vi "Histogram Matching.vi"() -> ()   [LabVIEW 2014]
doc: "Use this template to build a VI to use as a subVI."
uses:
  <vilib>/vision/NI_Vision_Development_Module.lvlib
panel:
  out "H-Target":T1(graph)
  out "Target":T2(plugin-control)
  out "H-Dst":T1(graph)
  out "Dst":T2(plugin-control)
  out "H-Src":T1(graph)
  out "Src":T2(plugin-control)
  # ":: MVi Framework V1.0 ::\nAuthor:Gaoke Yang\nEmail: gaoke.yang@yahoo.com\nWeb: www.mvicontrol.com\nCopyright (C) 2015, MVI Technologies All Rights Reserved"
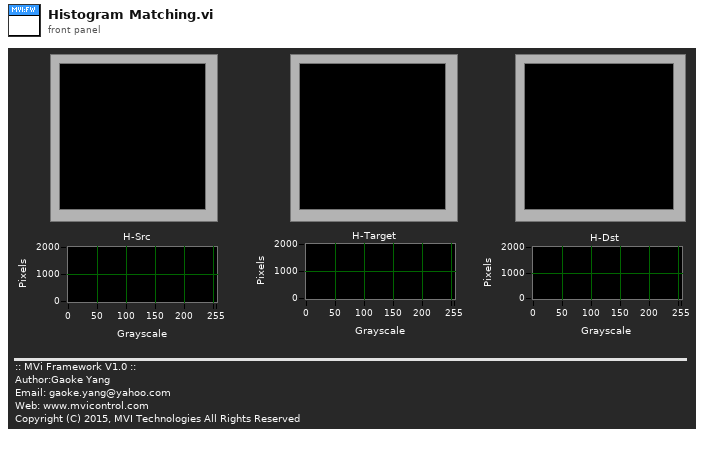
[diagram p1: front panel]
types:
  T1 = cluster{"Starting Value":sgl, "Incremental Value":sgl, "Histogram":u32[]}
  T2 = typedef "IMAQ Image.ctl" = refnum<image>
  T3 = typedef "Image Type" = u32
  T4 = cluster{"histogram":u32[], "Minimal Value":sgl, "Maximal Value":sgl, "Starting Value":sgl, "Interval Width":sgl, "Mean Value":sgl, "Standard  Variation":sgl, "Area (pixels)":i32}
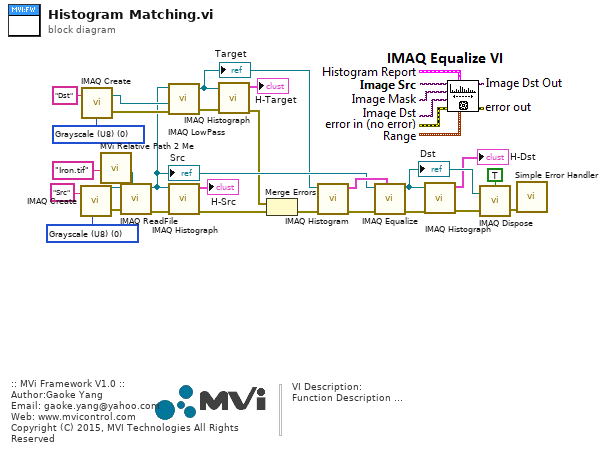
[diagram p0: block diagram]
diagram:
  w7 = T3 0 items=["Grayscale (U8)", "Grayscale (I16)", "Grayscale (SGL)", "Complex (CSG)", "RGB (U32)", "HSL (U32)", "RGB (U64)", "Grayscale (U16)"] ("Image Type")
  w12 = T3 0 items=["Grayscale (U8)", "Grayscale (I16)", "Grayscale (SGL)", "Complex (CSG)", "RGB (U32)", "HSL (U32)", "RGB (U64)", "Grayscale (U16)"] ("Image Type")
  # "VI Description:\nFunction Description ..."
  # ":: MVi Framework V1.0 ::\nAuthor:Gaoke Yang\nEmail: gaoke.yang@yahoo.com\nWeb: www.mvicontrol.com\nCopyright (C) 2015, MVI Technologies All Rights Reserved"
  n1 = call "IMAQ Create"("Image Name"="Src" ("name or relative path"), "Image Type"=w12) -> ("New Image"=w22:T2, "error out"=w21:errorcluster)  [unwired: 2 in, 1 out]
  n2 = call "IMAQ Create"("Image Name"="Dst" ("name or relative path"), "Image Type"=w7) -> ("New Image"=w6:T2, "error out"=w11:errorcluster)  [unwired: 2 in, 1 out]
  n3 = call "MVi Relative Path 2 Me.vi"("Relative Path"="Iron.tif" ("name or relative path")) -> ("Appended Dir"=w23:path)  [unwired: 5 in, 1 out]
  n4 = call "IMAQ ReadFile"("File Path"=w23, "error in (no error)"=w21, "Image"=w22) -> ("error out"=w20:errorcluster, "Image Out"=w5:T2)  [unwired: 4 in, 3 out]
  "Src" <- w5
  n5 = call "IMAQ LowPass"("Image Src"=w5, "Image Dst"=w6, "error in (no error)"=w11) -> ("Image Dst Out"=w4:T2, "error out"=w9:errorcluster)  [unwired: 4 in]
  "Target" <- w4
  n6 = call "IMAQ Histograph"("error in (no error)"=w20, "Image"=w5) -> ("error out"=w2:errorcluster, "Histogram Graph"=→"H-Src":T1)  [unwired: 6 in, 2 out]
  n7 = call "IMAQ Histograph"("error in (no error)"=w9, "Image"=w4) -> ("error out"=w3:errorcluster, "Histogram Graph"=→"H-Target":T1)  [unwired: 6 in, 2 out]
  n8 = Merge Errors(w3, w2) -> (w1:errorcluster)
  n9 = call "IMAQ Histogram"("error in (no error)"=w1, "Image"=w4) -> ("error out"=w18:errorcluster, "Histogram Report"=w10:T4)  [unwired: 8 in]
  n10 = call "IMAQ Equalize"("Histogram Report"=w10, "error in (no error)"=w18, "Image Src"=w5) -> ("error out"=w17:errorcluster, "Image Dst Out"=w15:T2)  [unwired: 7 in]
  "Dst" <- w15
  n11 = call "IMAQ Histograph"("error in (no error)"=w17, "Image"=w15) -> ("error out"=w16:errorcluster, "Histogram Graph"=→"H-Dst":T1)  [unwired: 6 in, 2 out]
  n12 = call "IMAQ Dispose"("All Images? (No)"=TRUE, "Image"=w15, "error in (no error)"=w16) -> ("error out"=w24:errorcluster)  [unwired: 3 out]
  n13 = call <vilib>:"Simple Error Handler.vi"("error in (no error)"=w24) -> ()  [unwired: 1 in, 8 out]
